vi "WaveformAnalysis.vi"() -> ()   [LabVIEW 2009]
panel:
  out "Array":u8[](array[numeric])=[224, 224, 128, 28, 96, 84, 0, 0, 0, 0, 128, 0, 184, 0, 130, 0, 130, 0, 36, 3, 8, 0, 254, 254, 1, 192, 104, 46, 227, 224, 128, 24, 96, 86, 0, 0, 0, 0, 128, 0, 184, 0, 130, 0, 130, 0, 32, 2, 13, 0, 254, 254, 0, 192, 104, 46, 226] format="%.0x"
  out "Waveform Chart":waveform(dbl)(graph)={"t0"=timestamp(0 s since 1904-01-01), "dt"=4e-08, "Y"=array[499999 elements]}
  out "deleted portion 2":dbl[](array[numeric])
  out "deleted portion":dbl[](array[numeric])
  in  "all rows":dbl[][](array[numeric])=array500016x3[1500048 elements] format="%0.3f"
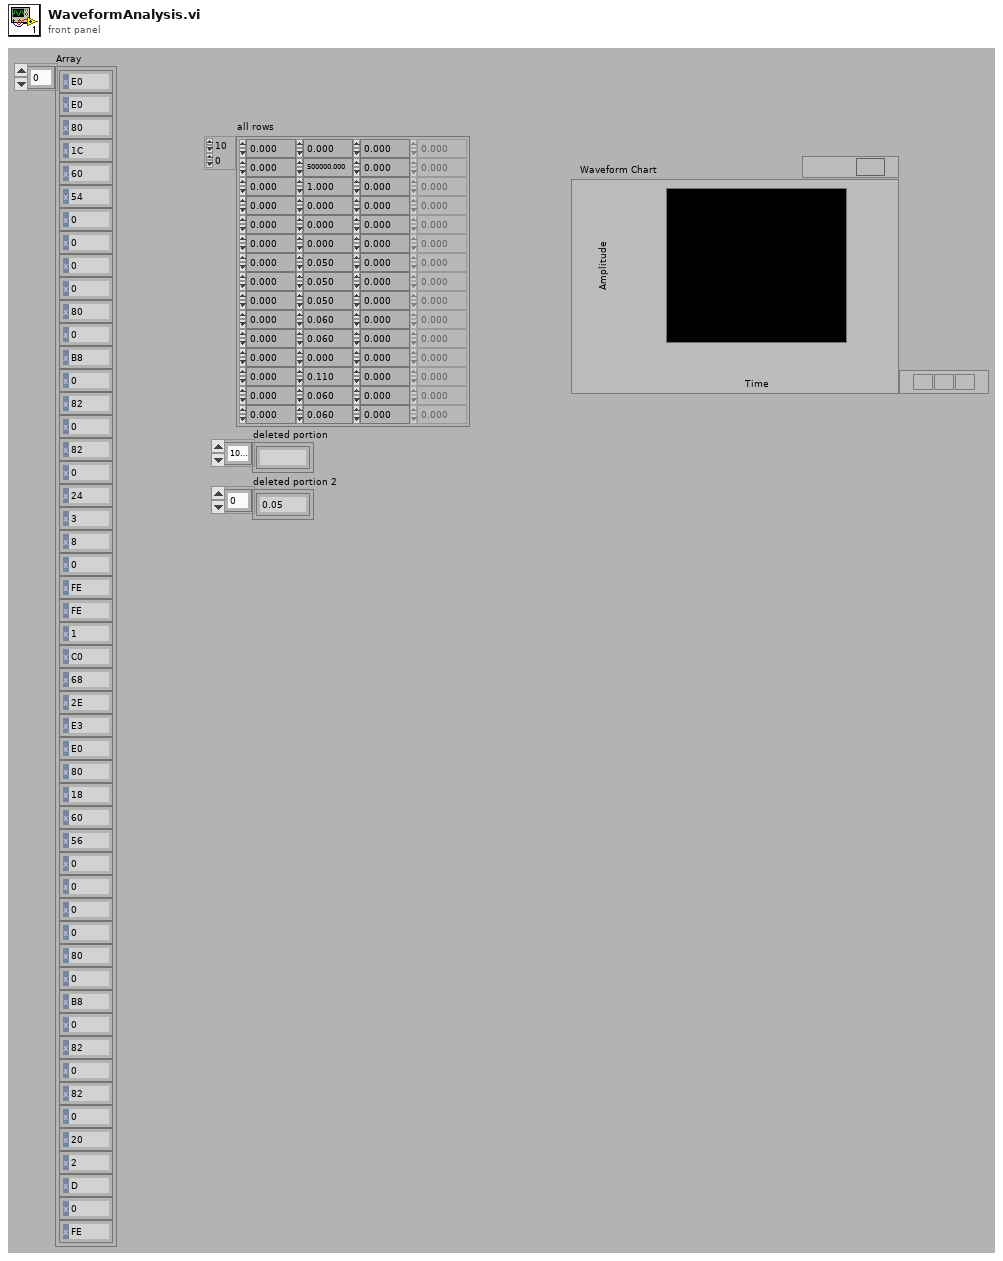
[diagram p1: front panel]
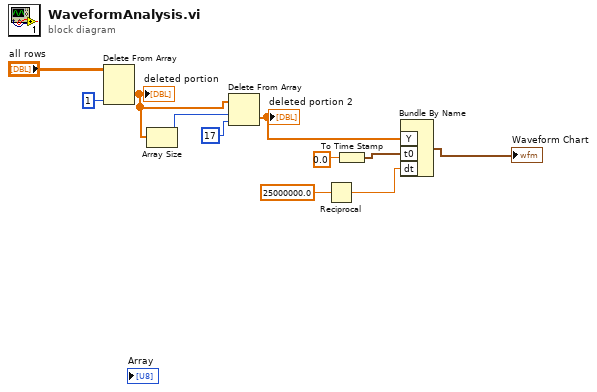
[diagram p0: block diagram]
diagram:
  n1 = Delete From Array(array="all rows", index (col)=1 ("disabled index (col)")) -> (deleted portion=w8:dbl[])  [unwired: 2 in, 1 out]
  "deleted portion" <- w8
  n2 = Array Size(array=w8) -> (size(s)=w7:i32)
  n3 = Delete From Array(array=w8, length=w7, index=17) -> (deleted portion=w6:dbl[])  [unwired: 1 out]
  "deleted portion 2" <- w6
  n4 = Reciprocal(x=25000000.0) -> (1/x=w3:dbl)
  n5 = To Time Stamp(1:0.0 ("disabled index (col)")) -> (0:w5:timestamp)
  n6 = Bundle By Name("Y"=w6, "t0"=w5, "dt"=w3) -> (→"Waveform Chart":waveform(dbl))  [unwired: 1 in]
